vi "HT Light.vi"(0 "I2C Ref In":T1={"myRIO Reference"={"myRIO Model"=enum."Unknown", "myRIO Hardware Reference"={"Generic FPGA Reference"=refnum, "Allow multiple opens"=FALSE}}, "I2C Channels Enum"=enum."Not Connected", "I2C Configuration"={"I2C Transfer Rate"=enum."Fast mode (400 kbps)"}}, 5 "Data Red":u8[](array[numeric])=[48], 7 "Data Green":u8[](array[numeric])=[48], 9 "Data Blue":u8[](array[numeric])=[48], 11 "error in (no error)":errorcluster, 13 "Address":u8=1 format="%x") -> (4 "I2C Ref Out":T1={"myRIO Reference"={"myRIO Model"=enum."Unknown", "myRIO Hardware Reference"={"Generic FPGA Reference"=refnum, "Allow multiple opens"=FALSE}}, "I2C Channels Enum"=enum."Not Connected", "I2C Configuration"={"I2C Transfer Rate"=enum."Fast mode (400 kbps)"}}, 6 "Red":u8, 8 "Green":u8, 10 "Blue":u8, 14 "error out":errorcluster, 15 "White":u8)   [LabVIEW 2017]
uses:
  <vilib>/myRIO/Instrument Drivers/Onboard IO/I2C/typedefs/I2C Reference.ctl
  <vilib>/myRIO/Common/Instrument Driver Framework/Utilities/typedefs/myRIO Generic Hardware Reference.ctl
  <vilib>/myRIO/Common/Instrument Driver Framework/Utilities/typedefs/Hardware Version Enum.ctl
  <vilib>/myRIO/Common/Instrument Driver Framework/Utilities/typedefs/myRIO v1.0 Reference.ctl
  <vilib>/myRIO/Common/Instrument Driver Framework/Utilities/typedefs/Generic FPGA Reference.ctl
  <vilib>/myRIO/Common/Instrument Driver Framework/myRIO v1.0/I2C/typedefs/I2C Channels Enum.ctl
  <vilib>/myRIO/Instrument Drivers/Onboard IO/I2C/typedefs/I2C Configuration.ctl
  <vilib>/myRIO/Instrument Drivers/Onboard IO/I2C/typedefs/I2C Transfer Rate.ctl
  <vilib>/Utility/error.llb/Error Cluster From Error Code.vi
  <vilib>/myRIO/Common/Instrument Driver Framework/myRIO v1.0/I2C/vis/myRIO v1.0 Write I2C.vi
  <vilib>/myRIO/Common/Instrument Driver Framework/myRIO v1.0/I2C/vis/myRIO v1.0 Read I2C.vi
  <vilib>/myRIO/Instrument Drivers/Onboard IO/I2C/I2C.lvlib
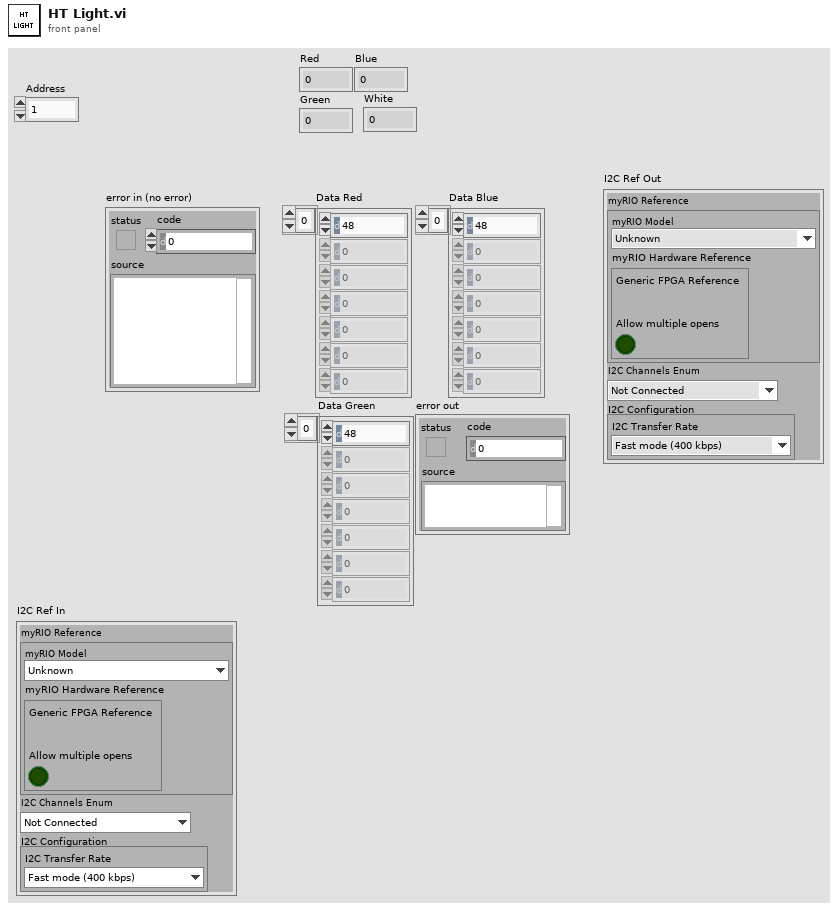
[diagram p1: front panel]
types:
  T1 = typedef "I2C.lvlib/I2C Reference.ctl" = cluster{"myRIO Reference":T2, "I2C Channels Enum":T6, "I2C Configuration":T7}
  T2 = typedef "myRIO Generic Hardware Reference.ctl" = cluster{"myRIO Model":T3, "myRIO Hardware Reference":T4}
  T3 = typedef "Hardware Version Enum.ctl" = enum16{"Unknown", "myRIO-1900", "myRIO-1950", "roboRIO", "NI ELVIS RIO CM"}
  T4 = typedef "myRIO v1.0 Reference.ctl" = cluster{"Generic FPGA Reference":T5, "Allow multiple opens":bool}
  T5 = typedef "Generic FPGA Reference.ctl" = refnum<k20>
  T6 = typedef "I2C Channels Enum.ctl" = enum16{"Not Connected", "A/I2C", "B/I2C", "I2C/I2C"}
  T7 = typedef "I2C.lvlib/I2C Configuration.ctl" = cluster{"I2C Transfer Rate":T8}
  T8 = typedef "I2C.lvlib/I2C Transfer Rate.ctl" = enum16{"Standard mode (100 kbps)", "Fast mode (400 kbps)"}
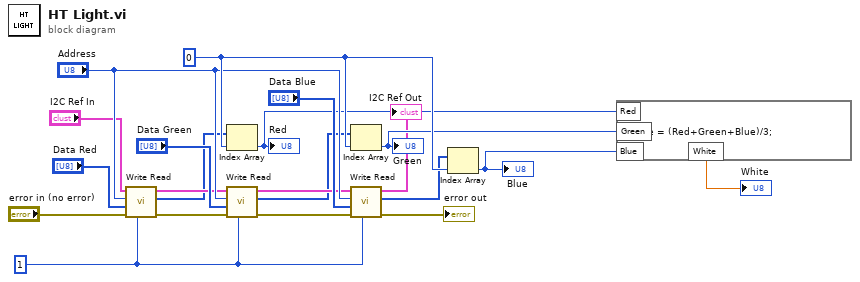
[diagram p0: block diagram]
diagram:
  w2 = 1
  w21 = 0 ("index")
  n1 = call <vilib>:"Write Read.vi"("Byte Count"=w2, "error in (no error)"="error in (no error)", "Bytes to Write"="Data Red", "Slave Address (7-bit)"="Address", "I2C Ref In"="I2C Ref In") -> ("error out"=w17:errorcluster, "Bytes Read"=w4:u8[], "I2C Ref Out"=w12:T1)  [unwired: 3 in]
  n2 = Index Array(array=w4, index=w21) -> (element=w3:u8)
  "Red" <- w3
  n3 = call <vilib>:"Write Read.vi"("Byte Count"=w2, "error in (no error)"=w17, "Bytes to Write"="Data Green", "Slave Address (7-bit)"="Address", "I2C Ref In"=w12) -> ("error out"=w16:errorcluster, "Bytes Read"=w8:u8[], "I2C Ref Out"=w11:T1)  [unwired: 3 in]
  n4 = Index Array(array=w8, index=w21) -> (element=w7:u8)
  "Green" <- w7
  n5 = call <vilib>:"Write Read.vi"("Byte Count"=w2, "error in (no error)"=w16, "Bytes to Write"="Data Blue", "Slave Address (7-bit)"="Address", "I2C Ref In"=w11) -> ("error out"=→"error out":errorcluster, "Bytes Read"=w6:u8[], "I2C Ref Out"=→"I2C Ref Out":T1)  [unwired: 3 in]
  n6 = Index Array(array=w6, index=w21) -> (element=w5:u8)
  "Blue" <- w5
  n7 = formula code="White = (Red+Green+Blue)/3;"("Red"=w3, "Green"=w7, "Blue"=w5) -> ("White"=→"White":dbl)
